vi "VITree.vi"   [LabVIEW 2017]
uses:
  Type Defs/Display Format.ctl
  Serializer.lvclass
  Serializer.JSON/Serializer.JSON.lvclass
  \\192.168.1.40\Neosoft/Partage/Dossiers Personnels/BRO/DevTools_BR/wc/ErrorLog/src/Serializer/Serializer.lvclass
  Serializer.PlainText/Serializer.PlainText.lvclass
  Serializer.PlainText.INI/Serializer.PlainText.INI.lvclass
  Serializer.XML/Serializer.XML.lvclass
  Serializer.lvlib
types:
  T1 = typedef "Serializer.lvlib/Display Format.ctl" = enum16{"PlainText", "PlainText.INI", "XML", "JSON"}
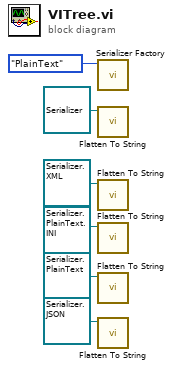
[diagram p0: block diagram]
diagram:
  n1 = call "Serializer Factory.vi"("Display Format"=Display_Format."PlainText") -> ()  [unwired: 9 in, 2 out]
  n2 = call "Flatten To String.vi"("Serializer in"=refnum<class "Serializer.lvclass"> refnum) -> ()  [unwired: 8 in, 3 out]
  n3 = call "Flatten To String.vi"("Serializer in"=refnum<class "Serializer.XML.lvclass"> refnum ("Serializer.Plug-in.lvlib:Serializer.XML.lvclass")) -> ()  [unwired: 8 in, 3 out]
  n4 = call "Flatten To String.vi"("Serializer in"=refnum<class "Serializer.PlainText.INI.lvclass"> refnum ("Serializer.Plug-in.lvlib:Serializer.PlainText.INI.lvclass")) -> ()  [unwired: 8 in, 3 out]
  n5 = call "Flatten To String.vi"("Serializer in"=refnum<class "Serializer.PlainText.lvclass"> refnum ("Serializer.Plug-in.lvlib:Serializer.PlainText.lvclass")) -> ()  [unwired: 8 in, 3 out]
  n6 = call "Flatten To String.vi"("Serializer in"=refnum<class "Serializer.JSON.lvclass"> refnum ("Serializer.Plug-in.lvlib:Serializer.JSON.lvclass")) -> ()  [unwired: 8 in, 3 out]
